vi "Read Config File Path.vi"(8 "error in (no error)":errorcluster, 11 "Configuration File In":refnum<class "Configuration File.lvclass">) -> (0 "error out":errorcluster, 2 "Config File Path":path, 3 "Configuration File Out":refnum<class "Configuration File.lvclass">)   [LabVIEW 2020, in "Configuration File.lvclass"]
doc: "Abstract method for reading the path of the configuration file. This method must be implemented in the class implementing the interface."
uses:
  Configuration File.lvclass
  Base/Base.lvclass
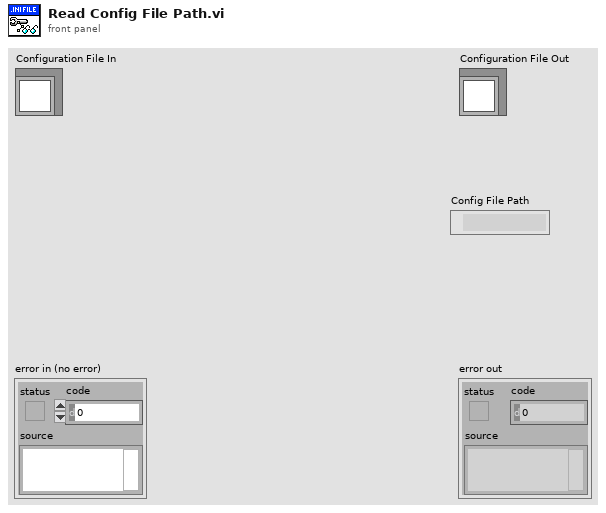
[diagram p1: front panel]
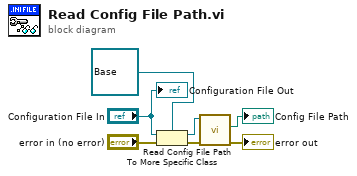
[diagram p0: block diagram]
diagram:
  n1 = To More Specific Class(target class=refnum<class "Base.lvclass"> refnum ("Base.lvclass"), reference="Configuration File In", error in="error in (no error)") -> (specific class reference=w6:refnum<class "Base.lvclass">, error out=w5:errorcluster)
  n2 = call "Read Config File Path.vi"("error in (no error)"=w5, "Process In"=w6) -> ("error out"=→"error out":errorcluster, "Config File Path"=→"Config File Path":path)  [unwired: 7 in, 1 out]
  "Configuration File Out" <- "Configuration File In"
